vi "Sensor_Reads.vi"() -> ()   [LabVIEW 2019]
uses:
  Globals/Drive_Globals.vi
  Globals/Flywheel_Globals.vi
  Globals/Control_Panel_Globals.vi
  Globals/Turret_Globals.vi
  Globals/Magazine_Globals.vi
  Globals/Sensor_Values.vi
  <vilib>/Rock Robotics/Network Tables/NT Read Number.vi
  Globals/Climb_Globals.vi
  <vilib>/Rock Robotics/WPI/ThirdParty/Phoenix-LabVIEW/Pigeon IMU/CTRE_PigeonIMU_GetYPR.vi
  <vilib>/Rock Robotics/WPI/ThirdParty/Phoenix-LabVIEW/Motor Controller/Get/CTRE_Phoenix_MotorController_GetSelectedSensorData.vi
panel:
  out "Magazine Position (Raw Sensor Units)":i32
  out "Sensor Position":dbl
  out "Climb_Top_Limit":bool
  out "Climb_Bottom_Limit":bool=TRUE
  in  "Top_IR_Threshold":dbl=1.0
  in  "Bottom_Middle_IR_Threshold":dbl=1.0
  in  "Top_Middle_IR_Threshold":dbl=1.0
  in  "Bottom_IR_Threshold":dbl=1.0
  out "Top_IR":bool
  out "Bottom_Middle_IR":bool
  out "Top_Middle_IR":bool
  out "Bottom_IR":bool
  out "Top_IR_Voltage":dbl
  out "Top_Middle_IR_Voltage":dbl
  out "Bottom_Middle_IR_Voltage":dbl
  out "Bottom_IR_Voltage":dbl
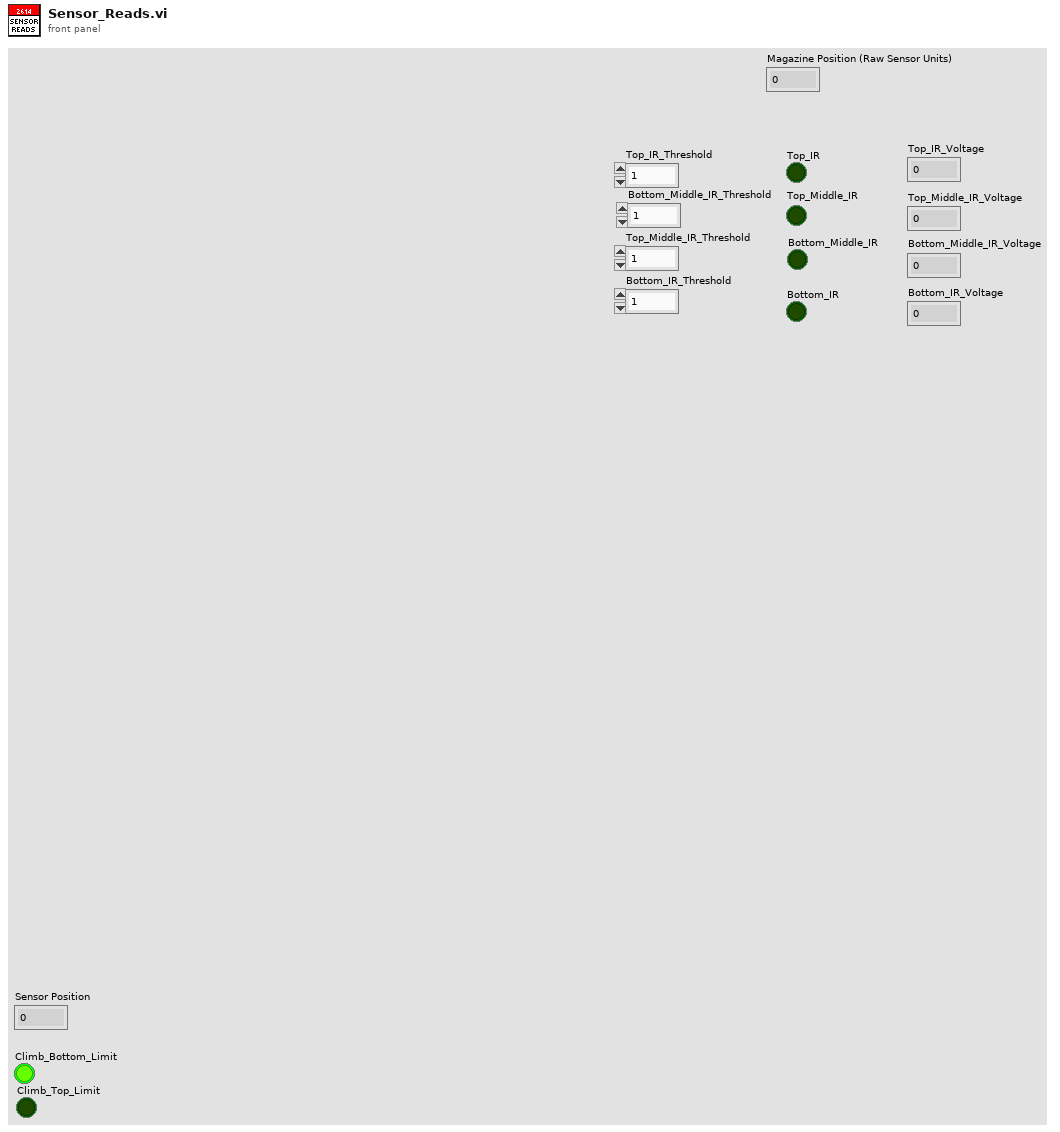
[diagram p1: front panel]
types:
  T1 = typedef "WPI_DigitalInputDevRef.ctl" = cluster{"DevStatus":errorcluster, "DIO Channel":T2}
  T2 = typedef "FPGA_DIOChannel.ctl" = enum8{"DIO 0", "DIO 1", "DIO 2", "DIO 3", "DIO 4", "DIO 5", "DIO 6", "DIO 7", "DIO 8", "DIO 9", "DIO MXP 0", "DIO MXP 1", "DIO MXP 2", "DIO MXP 3", "DIO MXP 4", "DIO MXP 5", "DIO MXP 6", "DIO MXP 7", "DIO MXP 8", "DIO MXP 9", "DIO MXP 10", "DIO MXP 11", "DIO MXP 12", "DIO MXP 13", "DIO MXP 14", "DIO MXP 15", "SPI Port CS1", "SPI Port CS2", "SPI Port CS3", "SPI Port MISO", "SPI Port MOSI", "Invalid"}
  T3 = typedef "WPI_MotorControlDeviceRef.ctl" = cluster{"DeviceStatus":errorcluster, "Type":T4, "PWM":cluster{"PWM Channel":T5, "DeadBand":T6}, "CAN":cluster{"Device Number":u8, "SetOutput VI Ref":variant, "GetOutput VI Ref":variant, "Enable VI Ref":variant, "Disable VI Ref":variant, "Data":variant}, "Invert":bool, "DIO PWM":cluster{"PWM \"Enable\" Channel":T5, "DIOChannel":T2, "PWM Rate":dbl}}
  T4 = typedef "WPI_MotorControlType.ctl" = enum16{"PWM", "CAN", "DIO PWM"}
  T5 = typedef "FPGA_DIOPWMChannel.ctl" = enum8{"PWM 0", "PWM 1", "PWM 2", "PWM 3", "PWM 4", "PWM 5", "PWM 6", "PWM 7", "PWM 8", "PWM 9", "PWM MXP 0", "PWM MXP 1", "PWM MXP 2", "PWM MXP 3", "PWM MXP 4", "PWM MXP 5", "PWM MXP 6", "PWM MXP 7", "PWM MXP 8", "PWM MXP 9", "Invalid"}
  T6 = typedef "WPI_PWMDeadband.ctl" = cluster{"Name":string, "maxPositivePwm":i32, "minPositivePwm":i32, "centerPwm":i32, "maxNegativePwm":i32, "minNegativePwm":i32, "angularRange":u16}
  T7 = typedef "CTRE_PigeonIMU_DeviceRef.ctl" = cluster{"DeviceStatus":errorcluster, "Device Number":u8, "Type":T8, "Device ID":u32, "Handle":u64, "UsageFrame":u32, "Library Path":path}
  T8 = typedef "CTRE_PigeonIMU_ConnectionType.ctl" = u32
  T9 = typedef "WPI_AnalogChannelDevRef.ctl" = cluster{"DevStatus":errorcluster, "Analog Channel":T10}
  T10 = typedef "FPGA_AIChannel.ctl" = enum8{"AI 0", "AI 1", "AI 2", "AI 3", "AI MXP 0", "AI MXP 1", "AI MXP 2", "AI MXP 3", "Invalid"}
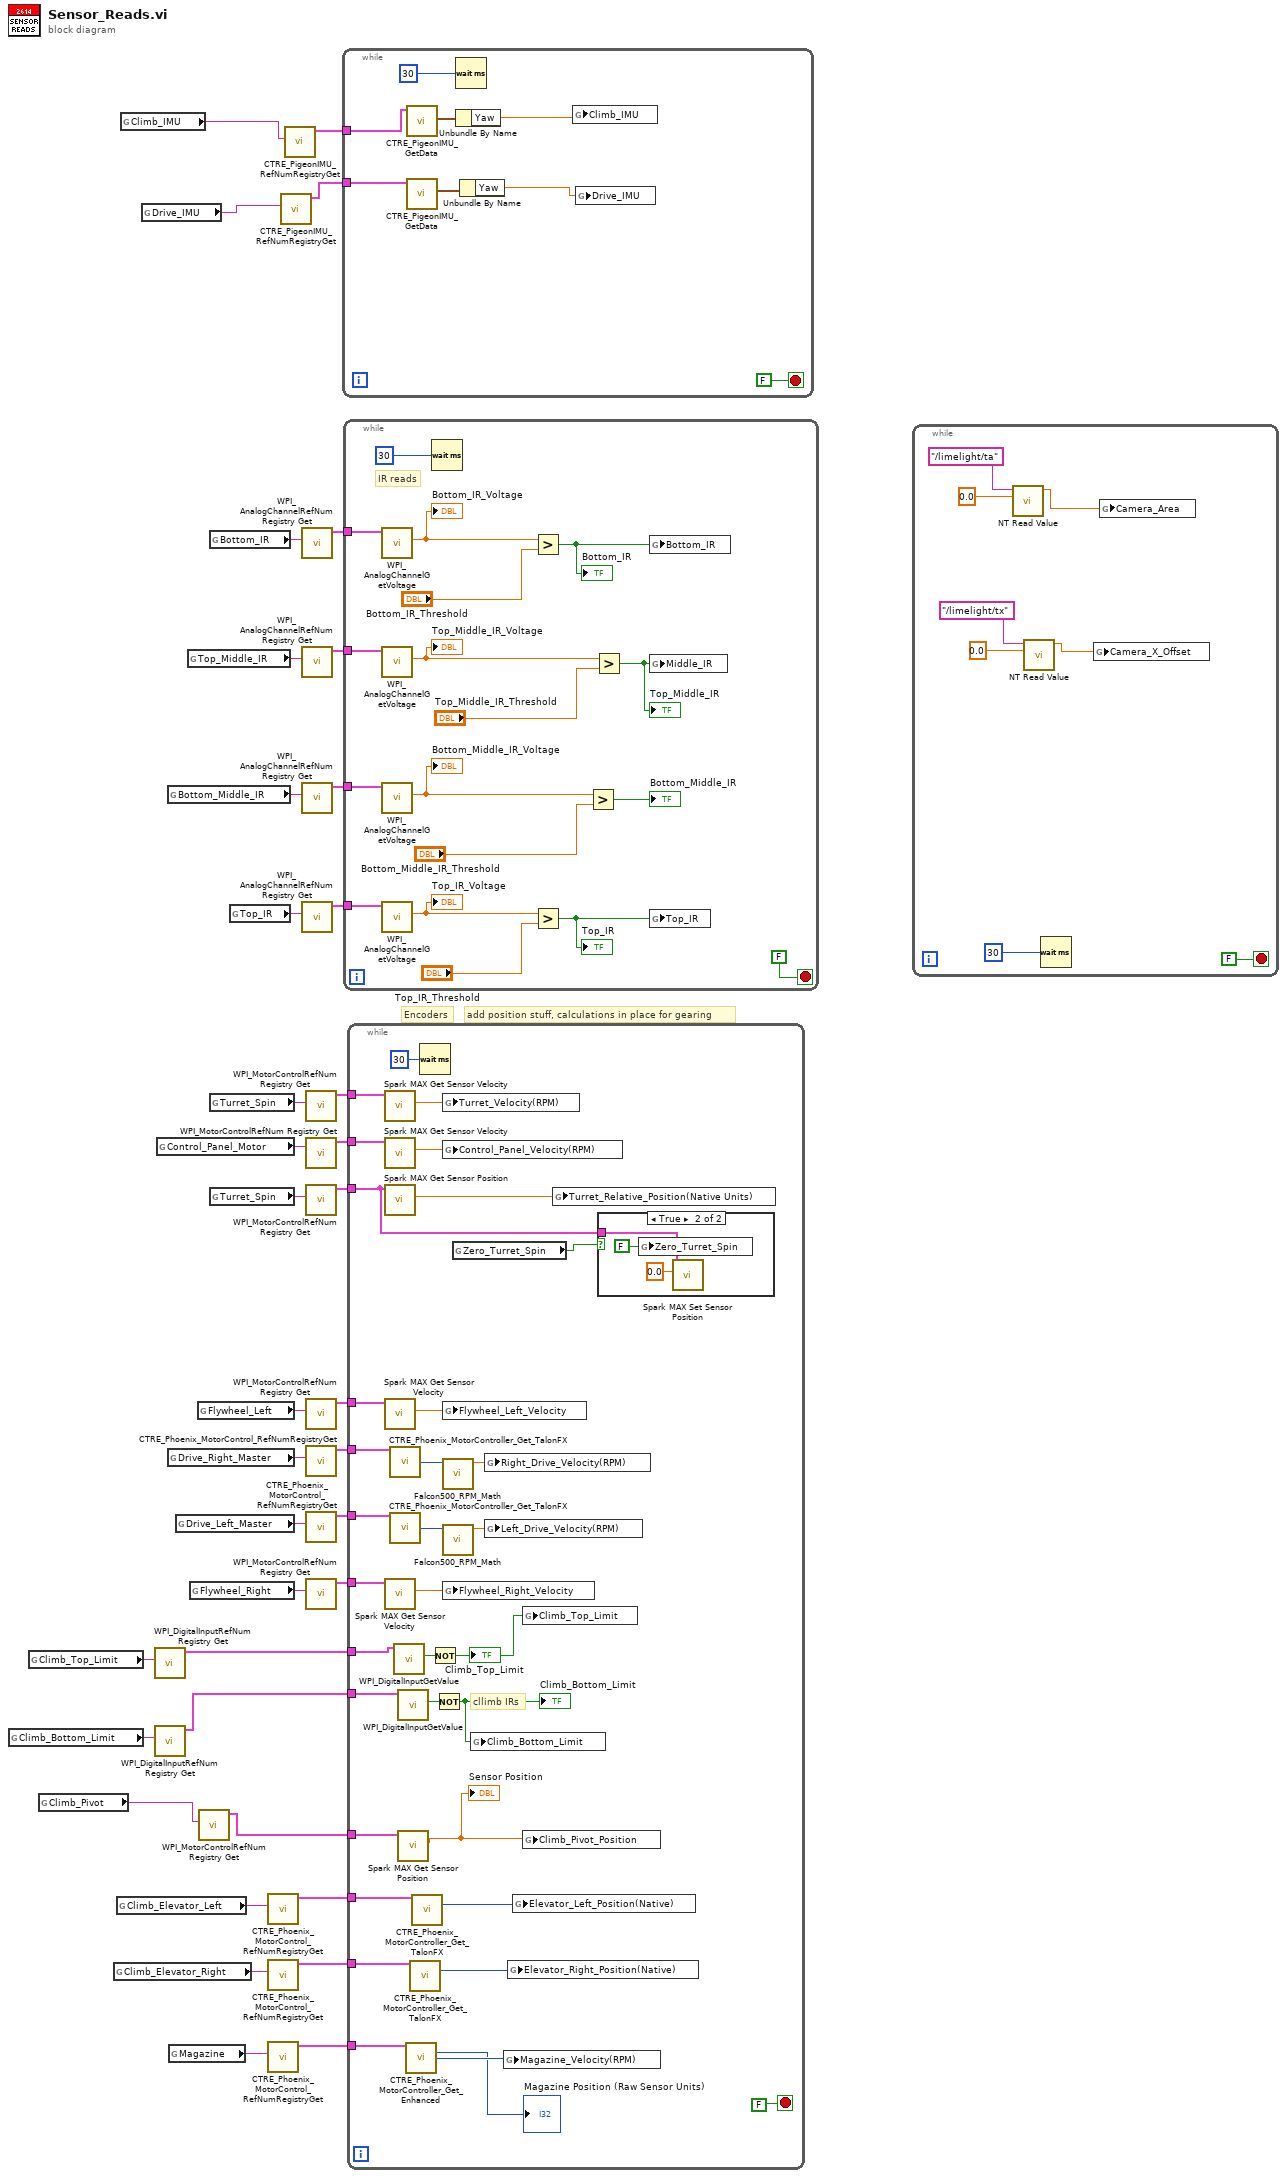
[diagram p0: block diagram]
diagram:
  # "add position stuff, calculations in place for gearing"
  # "Encoders"
  n1 = global read "Climb_Globals.vi" "Climb_Bottom_Limit"() -> (w15:string)
  n2 = global read "Climb_Globals.vi" "Climb_Top_Limit"() -> (w16:string)
  n3 = global read "Climb_Globals.vi" "Climb_Pivot"() -> (w14:string)
  n4 = global read "Climb_Globals.vi" "Climb_Elevator_Right"() -> (w9:string)
  n5 = global read "Climb_Globals.vi" "Climb_Elevator_Left"() -> (w10:string)
  n6 = global read "Climb_Globals.vi" "Climb_IMU"() -> (w4:string)
  n7 = global read "Drive_Globals.vi" "Drive_IMU"() -> (w3:string)
  n8 = call <vilib>:"WPI_DigitalInputRefNum Registry Get.vi"("refnum name"=w16) -> ("DigitalInputDevRef"=w12:T1)  [unwired: 9 in, 1 out]
  n9 = call <vilib>:"WPI_DigitalInputRefNum Registry Get.vi"("refnum name"=w15) -> ("DigitalInputDevRef"=w13:T1)  [unwired: 9 in, 1 out]
  n10 = global read "Control_Panel_Globals.vi" "Control_Panel_Motor"() -> (w30:string)
  n11 = global read "Magazine_Globals.vi" "Bottom_Middle_IR"() -> (w23:string)
  n12 = global read "Drive_Globals.vi" "Drive_Right_Master"() -> (w37:string)
  n13 = global read "Magazine_Globals.vi" "Magazine"() -> (w6:string)
  n14 = global read "Drive_Globals.vi" "Drive_Left_Master"() -> (w38:string)
  n15 = global read "Magazine_Globals.vi" "Top_Middle_IR"() -> (w22:string)
  n16 = global read "Flywheel_Globals.vi" "Flywheel_Right"() -> (w33:string)
  n17 = global read "Flywheel_Globals.vi" "Flywheel_Left"() -> (w34:string)
  n18 = call <vilib>:"WPI_MotorControlRefNum Registry Get.vi"("refnum name"=w14) -> ("MotorControlDevRef"=w11:T3)  [unwired: 9 in, 1 out]
  n19 = global read "Magazine_Globals.vi" "Bottom_IR"() -> (w24:string)
  n20 = global read "Turret_Globals.vi" "Turret_Spin"() -> (w28:string)
  n21 = global read "Turret_Globals.vi" "Turret_Spin"() -> (w26:string)
  n22 = global read "Magazine_Globals.vi" "Top_IR"() -> (w21:string)
  n23 = call <vilib>:"CTRE_Phoenix_MotorControl_RefNumRegistryGet.vi"("refnum name"=w10) -> ("PhoenixMotorControlDevRef"=w8:T3)  [unwired: 9 in, 1 out]
  n24 = call <vilib>:"CTRE_Phoenix_MotorControl_RefNumRegistryGet.vi"("refnum name"=w9) -> ("PhoenixMotorControlDevRef"=w7:T3)  [unwired: 9 in, 1 out]
  n25 = call <vilib>:"CTRE_Phoenix_MotorControl_RefNumRegistryGet.vi"("refnum name"=w6) -> ("PhoenixMotorControlDevRef"=w5:T3)  [unwired: 9 in, 1 out]
  n26 = call <vilib>:"CTRE_PigeonIMU_RefNumRegistryGet.vi"("refnum name"=w3) -> ("PigeonIMUDevRef"=w2:T7)  [unwired: 9 in, 1 out]
  n27 = call <vilib>:"CTRE_PigeonIMU_RefNumRegistryGet.vi"("refnum name"=w4) -> ("PigeonIMUDevRef"=w1:T7)  [unwired: 9 in, 1 out]
  n28 = call <vilib>:"WPI_AnalogChannelRefNum Registry Get.vi"("refnum name"=w24) -> ("AIDeviceRef"=w17:T9)  [unwired: 9 in, 1 out]
  n29 = call <vilib>:"WPI_AnalogChannelRefNum Registry Get.vi"("refnum name"=w22) -> ("AIDeviceRef"=w19:T9)  [unwired: 9 in, 1 out]
  n30 = call <vilib>:"WPI_AnalogChannelRefNum Registry Get.vi"("refnum name"=w23) -> ("AIDeviceRef"=w18:T9)  [unwired: 9 in, 1 out]
  n31 = call <vilib>:"WPI_AnalogChannelRefNum Registry Get.vi"("refnum name"=w21) -> ("AIDeviceRef"=w20:T9)  [unwired: 9 in, 1 out]
  n32 = call <vilib>:"WPI_MotorControlRefNum Registry Get.vi"("refnum name"=w28) -> ("MotorControlDevRef"=w27:T3)  [unwired: 9 in, 1 out]
  n33 = call <vilib>:"WPI_MotorControlRefNum Registry Get.vi"("refnum name"=w30) -> ("MotorControlDevRef"=w29:T3)  [unwired: 9 in, 1 out]
  n34 = call <vilib>:"WPI_MotorControlRefNum Registry Get.vi"("refnum name"=w26) -> ("MotorControlDevRef"=w25:T3)  [unwired: 9 in, 1 out]
  n35 = call <vilib>:"WPI_MotorControlRefNum Registry Get.vi"("refnum name"=w34) -> ("MotorControlDevRef"=w32:T3)  [unwired: 9 in, 1 out]
  n36 = call <vilib>:"CTRE_Phoenix_MotorControl_RefNumRegistryGet.vi"("refnum name"=w37) -> ("PhoenixMotorControlDevRef"=w36:T3)  [unwired: 9 in, 1 out]
  n37 = call <vilib>:"CTRE_Phoenix_MotorControl_RefNumRegistryGet.vi"("refnum name"=w38) -> ("PhoenixMotorControlDevRef"=w35:T3)  [unwired: 9 in, 1 out]
  n38 = call <vilib>:"WPI_MotorControlRefNum Registry Get.vi"("refnum name"=w33) -> ("MotorControlDevRef"=w31:T3)  [unwired: 9 in, 1 out]
  n39 = while {
    tunnel: w2 -> [w44]
    tunnel: w1 -> [w43]
    stop <- FALSE stop-if-true
    n40 = call-poly <vilib>:"CTRE_PigeonIMU_GetData.vi"("PigeonIMUDevRef"=w43) -> ("Yaw Pitch Roll"=w42:cluster{"Yaw":dbl, "Pitch":dbl, "Roll":dbl})  [unwired: 8 in, 2 out]
    n41 = call-poly <vilib>:"CTRE_PigeonIMU_GetData.vi"("PigeonIMUDevRef"=w44) -> ("Yaw Pitch Roll"=w41:cluster{"Yaw":dbl, "Pitch":dbl, "Roll":dbl})  [unwired: 8 in, 2 out]
    n42 = Wait (ms)(milliseconds to wait=u32 30) -> ()  [unwired: 1 out]
    n43 = Unbundle By Name(w42) -> ("Yaw"=w40:dbl)
    n44 = Unbundle By Name(w41) -> ("Yaw"=w39:dbl)
    n45 = global write "Sensor_Values.vi" "Climb_IMU"(w40) -> ()
    n46 = global write "Sensor_Values.vi" "Drive_IMU"(w39) -> ()
  }
  n47 = while {
    tunnel: w20 -> [w52]
    tunnel: w19 -> [w51]
    tunnel: w18 -> [w50]
    tunnel: w17 -> [w49]
    stop <- FALSE stop-if-true
    # "IR reads"
    n48 = call <vilib>:"WPI_AnalogChannelGetVoltage.vi"("AIDeviceRef"=w49) -> ("Voltage"=w60:dbl)  [unwired: 8 in, 2 out]
    "Bottom_IR_Voltage" <- w60
    n49 = call <vilib>:"WPI_AnalogChannelGetVoltage.vi"("AIDeviceRef"=w51) -> ("Voltage"=w58:dbl)  [unwired: 8 in, 2 out]
    "Top_Middle_IR_Voltage" <- w58
    n50 = call <vilib>:"WPI_AnalogChannelGetVoltage.vi"("AIDeviceRef"=w50) -> ("Voltage"=w59:dbl)  [unwired: 8 in, 2 out]
    "Bottom_Middle_IR_Voltage" <- w59
    n51 = call <vilib>:"WPI_AnalogChannelGetVoltage.vi"("AIDeviceRef"=w52) -> ("Voltage"=w53:dbl)  [unwired: 8 in, 2 out]
    "Top_IR_Voltage" <- w53
    n52 = Wait (ms)(milliseconds to wait=u32 30) -> ()  [unwired: 1 out]
    n53 = Greater?(x=w60, y="Bottom_IR_Threshold") -> (0:w64:bool)
    "Bottom_IR" <- w64
    n54 = Greater?(x=w53, y="Top_IR_Threshold") -> (0:w61:bool)
    "Top_IR" <- w61
    n55 = Greater?(x=w59, y="Bottom_Middle_IR_Threshold") -> (0:→"Bottom_Middle_IR":bool)
    n56 = Greater?(x=w58, y="Top_Middle_IR_Threshold") -> (0:w62:bool)
    "Top_Middle_IR" <- w62
    n57 = global write "Sensor_Values.vi" "Bottom_IR"(w64) -> ()
    n58 = global write "Sensor_Values.vi" "Middle_IR"(w62) -> ()
    n59 = global write "Sensor_Values.vi" "Top_IR"(w61) -> ()
  }
  n60 = while {
    tunnel: w36 -> [w97]
    tunnel: w35 -> [w96]
    tunnel: w32 -> [w90]
    tunnel: w31 -> [w89]
    tunnel: w29 -> [w87]
    tunnel: w27 -> [w85]
    tunnel: w25 -> [w80]
    tunnel: w13 -> [w74]
    tunnel: w12 -> [w73]
    tunnel: w11 -> [w72]
    tunnel: w8 -> [w71]
    tunnel: w7 -> [w70]
    tunnel: w5 -> [w67]
    stop <- FALSE stop-if-true
    # "cllimb IRs"
    n61 = call <vilib>:"Spark MAX Get Sensor Velocity.vi"("MotorControlDevRef in"=w85) -> ("Sensor Velocity"=w84:dbl)  [unwired: 7 in, 3 out]
    n62 = call <vilib>:"Spark MAX Get Sensor Velocity.vi"("MotorControlDevRef in"=w87) -> ("Sensor Velocity"=w86:dbl)  [unwired: 7 in, 3 out]
    n63 = call <vilib>:"Spark MAX Get Sensor Position.vi"("MotorControlDevRef in"=w80) -> ("Sensor Position"=w82:dbl)  [unwired: 7 in, 3 out]
    n64 = call <vilib>:"Spark MAX Get Sensor Velocity.vi"("MotorControlDevRef in"=w90) -> ("Sensor Velocity"=w83:dbl)  [unwired: 7 in, 3 out]
    n65 = call <vilib>:"Spark MAX Get Sensor Velocity.vi"("MotorControlDevRef in"=w89) -> ("Sensor Velocity"=w88:dbl)  [unwired: 7 in, 3 out]
    n66 = call-poly <vilib>:"CTRE_Phoenix_MotorController_Get_TalonFX.vi"("PhoenixMotorControlDevRef"=w97) -> ("Velocity (Raw Sensor Units per 100 ms)"=w95:i32)  [unwired: 11 in, 3 out]
    n67 = call-poly <vilib>:"CTRE_Phoenix_MotorController_Get_TalonFX.vi"("PhoenixMotorControlDevRef"=w96) -> ("Velocity (Raw Sensor Units per 100 ms)"=w93:i32)  [unwired: 11 in, 3 out]
    n68 = call <vilib>:"WPI_DigitalInputGetValue.vi"("DigitalInputDevRef"=w73) -> ("Value"=w79:bool)  [unwired: 8 in, 2 out]
    n69 = call <vilib>:"WPI_DigitalInputGetValue.vi"("DigitalInputDevRef"=w74) -> ("Value"=w77:bool)  [unwired: 8 in, 2 out]
    n70 = call <vilib>:"Spark MAX Get Sensor Position.vi"("MotorControlDevRef in"=w72) -> ("Sensor Position"=w75:dbl)  [unwired: 7 in, 3 out]
    "Sensor Position" <- w75
    n71 = call-poly <vilib>:"CTRE_Phoenix_MotorController_Get_Enhanced.vi"("PhoenixMotorControlDevRef"=w67) -> ("Position (Raw Sensor Units)"=→"Magazine Position (Raw Sensor Units)":i32, "Velocity (Raw Sensor Units per 100 ms)"=w66:i32)  [unwired: 11 in, 2 out]
    n72 = call-poly <vilib>:"CTRE_Phoenix_MotorController_Get_TalonFX.vi"("PhoenixMotorControlDevRef"=w70) -> ("Position (Raw Sensor Units)"=w68:i32)  [unwired: 11 in, 3 out]
    n73 = call-poly <vilib>:"CTRE_Phoenix_MotorController_Get_TalonFX.vi"("PhoenixMotorControlDevRef"=w71) -> ("Position (Raw Sensor Units)"=w69:i32)  [unwired: 11 in, 3 out]
    n74 = Wait (ms)(milliseconds to wait=u32 30) -> ()  [unwired: 1 out]
    n75 = Not(x=w79) -> (.not. x?=w76:bool)
    "Climb_Top_Limit" <- w76
    n76 = Not(x=w77) -> (.not. x?=w78:bool)
    "Climb_Bottom_Limit" <- w78
    n77 = global write "Sensor_Values.vi" "Turret_Velocity(RPM)"(w84) -> ()
    n78 = global write "Sensor_Values.vi" "Control_Panel_Velocity(RPM)"(w86) -> ()
    n79 = global write "Sensor_Values.vi" "Flywheel_Left_Velocity"(w83) -> ()
    n80 = call "Falcon500_RPM_Math.vi"("Velocity(native)"=w95) -> ("RPM"=w94:dbl)  [unwired: 10 in]
    n81 = call "Falcon500_RPM_Math.vi"("Velocity(native)"=w93) -> ("RPM"=w92:dbl)  [unwired: 10 in]
    n82 = global write "Sensor_Values.vi" "Flywheel_Right_Velocity"(w88) -> ()
    n83 = global read "Sensor_Values.vi" "Zero_Turret_Spin"() -> (w81:bool)
    n84 = global write "Sensor_Values.vi" "Climb_Bottom_Limit"(w78) -> ()
    n85 = global write "Sensor_Values.vi" "Right_Drive_Velocity(RPM)"(w94) -> ()
    n86 = global write "Sensor_Values.vi" "Left_Drive_Velocity(RPM)"(w92) -> ()
    n87 = global write "Sensor_Values.vi" "Magazine_Velocity(RPM)"(w66) -> ()
    n88 = global write "Sensor_Values.vi" "Elevator_Right_Position(Native)"(w68) -> ()
    n89 = global write "Sensor_Values.vi" "Elevator_Left_Position(Native)"(w69) -> ()
    n90 = global write "Sensor_Values.vi" "Climb_Top_Limit"(w76) -> ()
    n91 = global write "Sensor_Values.vi" "Climb_Pivot_Position"(w75) -> ()
    n92 = global write "Sensor_Values.vi" "Turret_Relative_Position(Native Units)"(w82) -> ()
    n93 = case shown="True" w81 {
      tunnel: w80 -> [_ w99]
      frame False {
      }
      frame True {
        n94 = global write "Sensor_Values.vi" "Zero_Turret_Spin"(FALSE ("Zero_Turret_Spin")) -> ()
        n95 = call <vilib>:"Spark MAX Set Sensor Position.vi"("Position"=0.0, "MotorControlDeviceRef"=w99) -> ()  [unwired: 8 in, 2 out]
      }
    }
  }
  n96 = while {
    stop <- FALSE stop-if-true
    n97 = call-poly <vilib>:"NT Read Value.vi"("Default Value"=0.0, "Name"="/limelight/ta") -> ("Numeric"=w102:dbl)  [unwired: 8 in, 1 out]
    n98 = call-poly <vilib>:"NT Read Value.vi"("Default Value"=0.0, "Name"="/limelight/tx") -> ("Numeric"=w105:dbl)  [unwired: 8 in, 1 out]
    n99 = Wait (ms)(milliseconds to wait=u32 30) -> ()  [unwired: 1 out]
    n100 = global write "Sensor_Values.vi" "Camera_X_Offset"(w105) -> ()
    n101 = global write "Sensor_Values.vi" "Camera_Area"(w102) -> ()
  }
